vi "Load Test Case Comments.vi"(8 "error in (no error)":errorcluster, 10 "File Contents":string[][](array[string]), 11 "LUnit Test Vector In":refnum<class "LUnit Test Vector.lvclass">) -> (0 "error out":errorcluster, 3 "LUnit Test Vector Out":refnum<class "LUnit Test Vector.lvclass">)   [LabVIEW 2020, in "LUnit Test Vector.lvclass"]
uses:
  LUnit Test Vector.lvclass
  LUnit Test Vector.lvclass/LUnit Test Vector.ctl
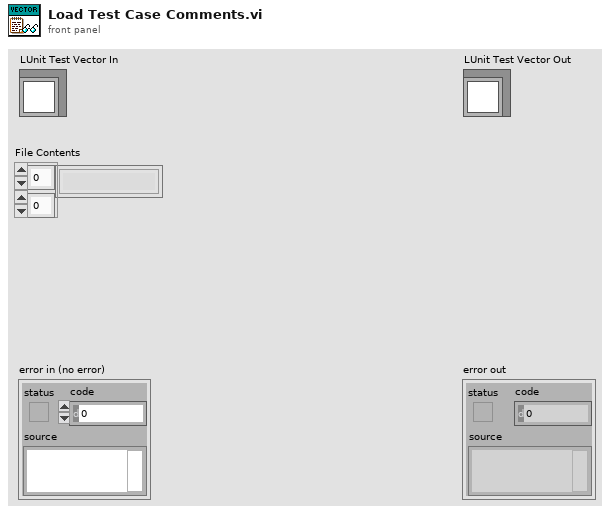
[diagram p1: front panel]
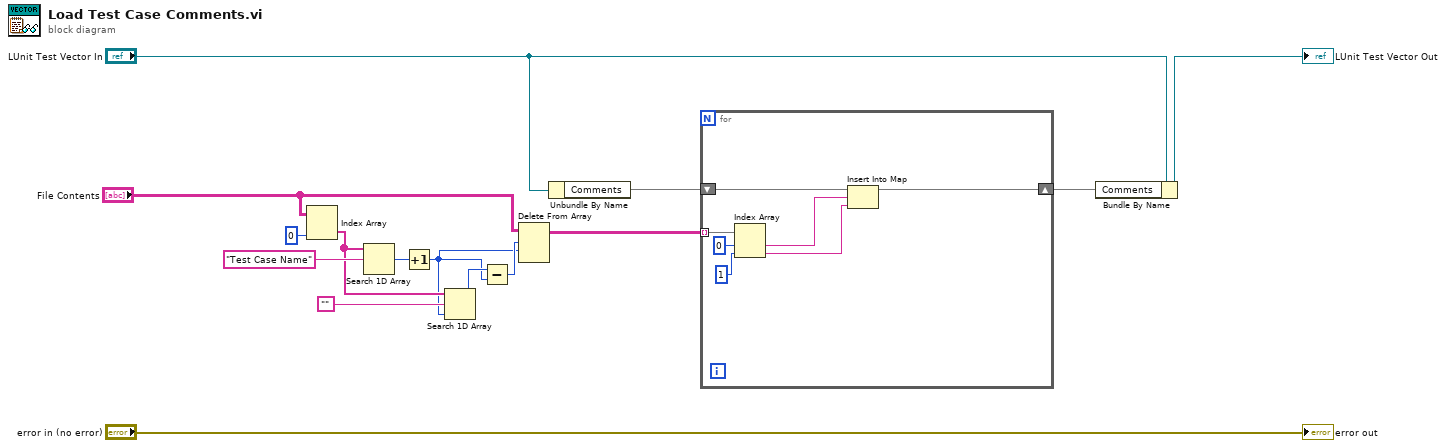
[diagram p0: block diagram]
diagram:
  n1 = Index Array(array="File Contents", index (col)=0 ("disabled index (col)")) -> (element=w11:string[])  [unwired: 1 in]
  n2 = Search 1D Array(1D array=w11, element="Test Case Name") -> (index of element=w9:i32)  [unwired: 1 in]
  n3 = Increment(x=w9) -> (x+1=w7:i32)
  n4 = Search 1D Array(1D array=w11, element="", start index (0)=w7) -> (index of element=w10:i32)
  n5 = Subtract(x=w10, y=w7) -> (x-y=w8:i32)
  n6 = Delete From Array(array="File Contents", length=w8, index (row)=w7) -> (array with subset deleted=w5:string[][])  [unwired: 1 in, 1 out]
  n7 = Unbundle By Name("LUnit Test Vector In") -> ("Comments"=w3:map{string, string})
  n8 = for {
    tunnel: w5 -> [w20] mode=indexing
    shift-right: [w21] -> w1
    shift-left: w3 -> [w22]
    n9 = Index Array(array=w20, index #1=0 ("index"), index #2=1 ("index")) -> (element #1=w17:string, element #2=w16:string)
    n10 = Insert Into Map(map in=w22, key=w17, value=w16) -> (map out=w21:map{string, string})  [unwired: 2 out]
  }
  n11 = Bundle By Name(cluster="LUnit Test Vector In", "Comments"=w1) -> (→"LUnit Test Vector Out":refnum<class "LUnit Test Vector.lvclass">)
  "error out" <- "error in (no error)"
